vi "Report_Type.vi"(8 "error in (no error)":errorcluster, 11 "IB_Source_Build in":refnum<class "IB_Source_Build.lvclass">) -> (0 "error out":errorcluster, 2 "type":string, 3 "IB_Source_Build out":refnum<class "IB_Source_Build.lvclass">)   [LabVIEW 2020, in "IB_Source_Build.lvclass"]
uses:
  <vilib>/AppBuilder/IB_Classes/Source/Container/Build/IB_Source_Build.lvclass
  <vilib>/AppBuilder/IB_Classes/Source/Container/Build/IB_Source_Build.lvclass/IB_Source_Build.ctl
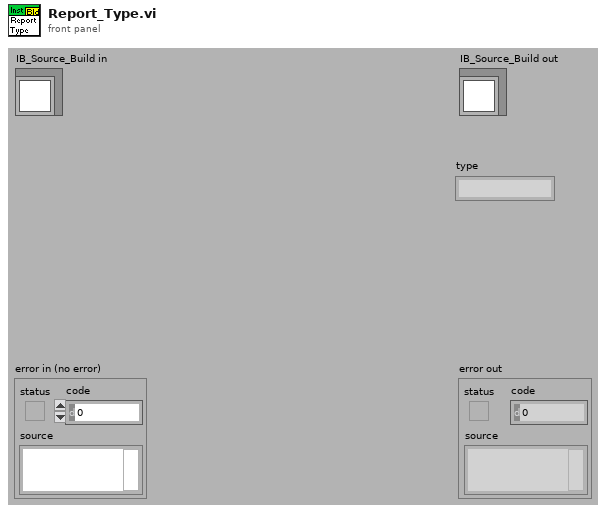
[diagram p1: front panel]
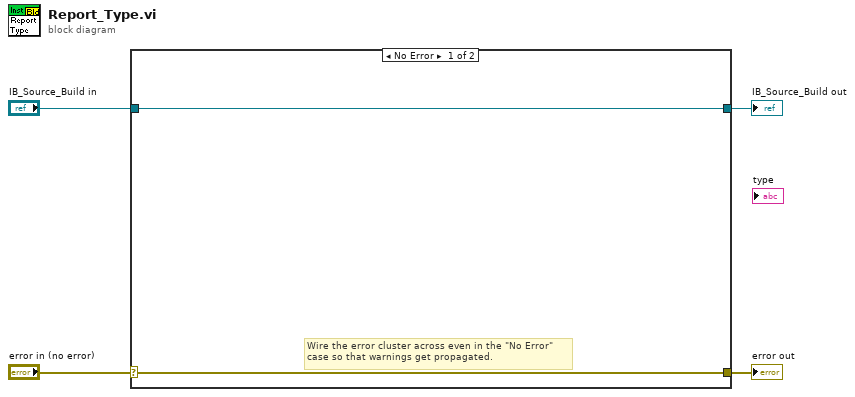
[diagram p0: block diagram]
diagram:
  n1 = case shown="No Error" "error in (no error)" {
    selector: "error in (no error)" -> [w5 w8]
    tunnel: [w5 w8] -> w3
    tunnel: [w6 w7] -> w1
    tunnel: "IB_Source_Build in" -> [w6 w7]
    frame No Error {
      # "Wire the error cluster across even in the \"No Error\"\ncase so that warnings get propagated."
    }
    frame Error {
    }
  }
  "error out" <- w3
  "IB_Source_Build out" <- w1
